vi "TypeConv_Register Existing Enums.vi"(10 "Enums":T1[](array[typedef]), 11 "Owning Lib":refnum<vi>) -> (3 "Owning Lib Dup":refnum<vi>)   [LabVIEW 2013]
uses:
  Action.ctl
  Category.ctl
  Data Structures/JSON/Enum Value.ctl
  Data Structures/JSON/Enum.ctl
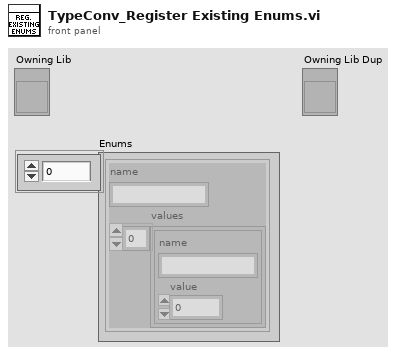
[diagram p1: front panel]
types:
  T1 = typedef "Enum.ctl" = cluster{"name":string, "values":T2[]}
  T2 = typedef "Enum Value.ctl" = cluster{"name":string, "value":i32}
  T3 = typedef "Category.ctl" = enum16{"Invalid", "Void", "Boolean", "Numeric", "Enum", "SimpleStruct", "OpaqueStruct", "SimpleIdentity", "QObject", "SimpleContainer", "FullArray"}
  T4 = typedef "Action.ctl" = enum16{"Register Type", "Register Projection", "Obtain Writer", "Get Projection"}
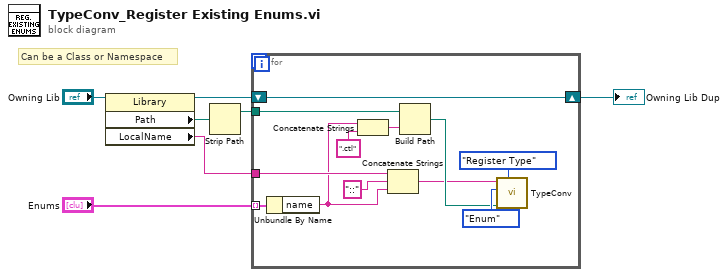
[diagram p0: block diagram]
diagram:
  # "Can be a Class or Namespace"
  n1 = property class="Library"(reference="Owning Lib") -> (reference out=w4:refnum<vi>, "Path"=w7:path, "LocalName"=w1:string)  [unwired: 1 in, 1 out]
  n2 = Strip Path(path=w7) -> (stripped path=w6:path)  [unwired: 1 out]
  n3 = for {
    tunnel: "Enums" -> [w19] mode=indexing
    tunnel: w6 -> [w17]
    shift-right: [w18] -> w3
    shift-left: w4 -> [w18]
    tunnel: w1 -> [w11]
    n4 = Unbundle By Name(w19) -> ("name"=w8:string)
    n5 = Concatenate Strings(w8, ".ctl" ("string")) -> (w15:string)
    n6 = Concatenate Strings(w11, "::" ("string"), w8) -> (w9:string)
    n7 = Build Path(base path=w17, name or relative path=w15) -> (appended path=w12:path)
    n8 = call "TypeConv.vi"("Action"=Action."Register Type", "Type Path"=w12, "Category"=Category."Enum", "Type Name"=w9) -> ()  [unwired: 7 in, 1 out]
  }
  "Owning Lib Dup" <- w3
